vi "ObtainQueue.vi"(7 "Destroy? (f)":bool, 8 "ErrorArray":errorcluster[](array[cluster])) -> (0 "ErrorArray.":errorcluster[](array[cluster]), 3 "TstQue":refnum<queue>)   [LabVIEW 2014, in "Test.lvclass"]
uses:
  Test.lvclass
  clQueMsgType.ctl
  <userlib>/NIST/NISTErrorLib/NISTErrorLib.lvlib
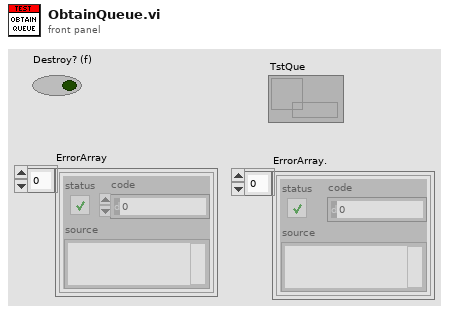
[diagram p1: front panel]
types:
  T1 = typedef "Test.lvclass/clQueMsgType.ctl" = cluster{"Message":string, "Data":variant}
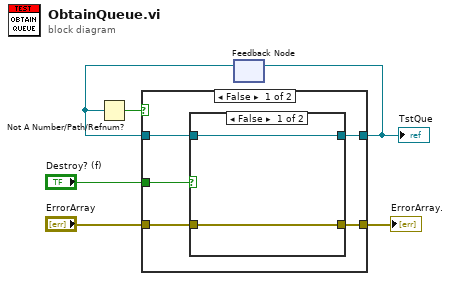
[diagram p0: block diagram]
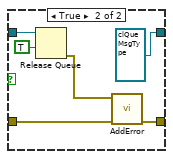
[diagram p2: hidden frame]
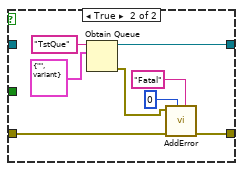
[diagram p3: hidden frame]
diagram:
  n1 = feedback #1() -> (w1:refnum<queue>)  [unwired: 1 in]
  n2 = Not A Number/Path/Refnum?(number/path/refnum=w1) -> (NaN/Path/Refnum?=w2:bool)
  n3 = case shown="False" w2 {
    tunnel: "ErrorArray" -> [w7 w25]
    tunnel: [w8 w22] -> w4
    tunnel: [w10 w20] -> w3
    tunnel: "Destroy? (f)" -> [w11 _]
    tunnel: w1 -> [w9 _]
    frame False {
      n4 = case shown="False" w11 {
        tunnel: w9 -> [w13 w19]
        tunnel: [w13 refnum<queue> refnum ("queue out")] -> w10
        tunnel: [w12 w15] -> w8
        tunnel: w7 -> [w12 w14]
        frame False {
        }
        frame True {
          n5 = Release Queue(queue=w19, force destroy? (F)=TRUE) -> (error out=w16:errorcluster)  [unwired: 1 in, 2 out]
          n6 = call <userlib>:"AddError.vi"("ErrorArray"=w14, "error in (no error)"=w16) -> ("ErrorArray"=w15:errorcluster[])  [unwired: 8 in, 1 out]
        }
      }
    }
    frame True {
      n7 = Obtain Queue(name (unnamed)="TstQue", element data type=T1 {"Message"="", "Data"=variant} ("clQueMsgType")) -> (queue out=w20:refnum<queue>, error out=w21:errorcluster)  [unwired: 3 in, 1 out]
      n8 = call <userlib>:"AddError.vi"("Severity"="Fatal", "Priority"=u8 0, "ErrorArray"=w25, "error in (no error)"=w21) -> ("ErrorArray"=w22:errorcluster[])  [unwired: 6 in, 1 out]
    }
  }
  "ErrorArray." <- w4
  "TstQue" <- w3
  n9 = feedback-in #1(w3) -> ()
